vi "Add Sub Address.vi"(0 "Remote Terminal in":refnum<k24>, 1 "SubAddress Config":T1 {"elapseMinOrMax" items=["A", "B", "AB", "None"]; "timeOrHitCount" items=["Time", "HitCount"]; "dataWipe" items=["Simulate", "Monitor", "Disable"]}, 5 "name":string, 7 "subAddress":i8, 9 "messageBufferIDRef (-1)":i32=-1, 11 "error in":errorcluster, 12 "direction (Tx)":i32(ring) items=["Tx", "Rx"]) -> (4 "Remote Terminal out":refnum<k24>, 6 "new Sub Address":refnum<k24>, 8 "ID out":i32, 15 "error out":errorcluster)   [LabVIEW 2020, in "Ballard_1553_Hardware_ni.lvlib"]
uses:
  Ballard_1553_Hardware_ni.lvlib
  C:/Users/Administrator/Desktop/GIT/Ballard-MIL-STD-1553-Custom-Device/Source/System Explorer/SubVIs/Parse XML Ballard/1.2/BTIXML_SerDes.dll
  Ballard-MIL-STD-1553-Custom-Device/Source/System Explorer/SubVIs/Parse XML Ballard/1.2/BTIXML_SerDes.dll
  _typedefs/subAddress_type.ctl
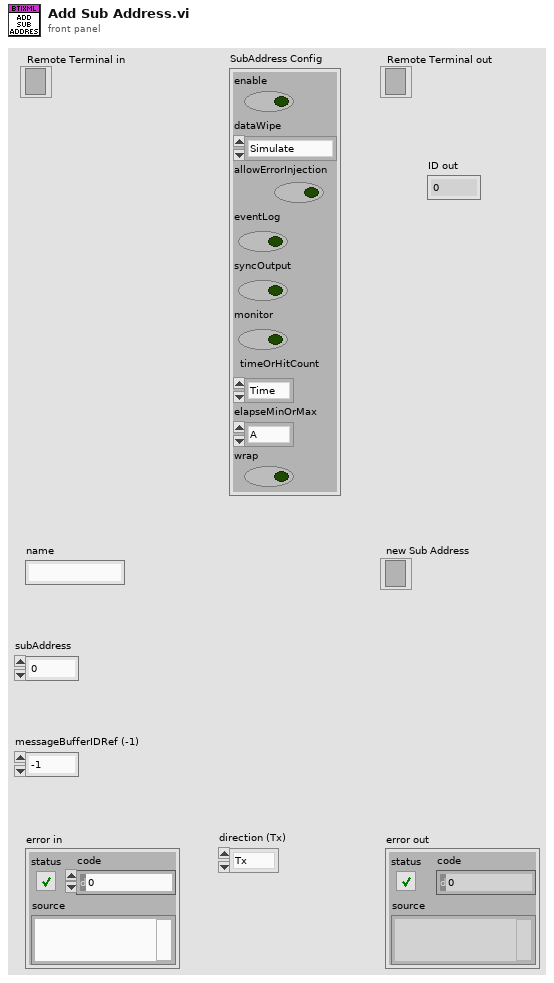
[diagram p1: front panel]
types:
  T1 = typedef "Ballard_1553_Hardware_ni.lvlib/subAddress_type.ctl" = cluster{"enable":bool, "dataWipe":i32, "allowErrorInjection":bool, "eventLog":bool, "syncOutput":bool, "monitor":bool, "timeOrHitCount":i32, "elapseMinOrMax":i32, "wrap":bool}
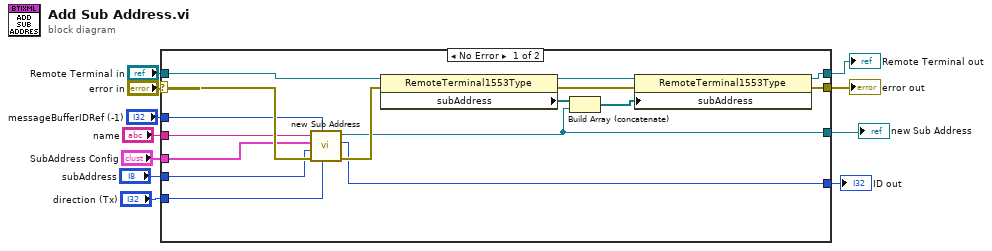
[diagram p0: block diagram]
diagram:
  n1 = case shown="No Error" "error in" {
    selector: "error in" -> [w20 w28]
    tunnel: [w25 w28] -> w11
    tunnel: [w26 w29] -> w8
    tunnel: "Remote Terminal in" -> [w27 w29]
    tunnel: [w18 _] -> w7
    tunnel: "messageBufferIDRef (-1)" -> [w17 _]
    tunnel: "name" -> [w16 _]
    tunnel: "SubAddress Config" -> [w15 _]
    tunnel: "direction (Tx)" -> [w14 _]
    tunnel: "subAddress" -> [w13 _]
    tunnel: [w12 _] -> w1
    frame No Error {
      n2 = call "new Sub Address.vi"("direction (Tx)"=w14, "messageBufferIDRef (-1)"=w17, "error in"=w20, "subAddress"=w13, "SubAddress Config"=w15, "name"=w16) -> ("error out"=w19:errorcluster, "ID out"=w12:i32, "subAddress out"=w18:refnum<k24>)  [unwired: 3 in]
      n3 = property class="RemoteTerminal1553Type"(reference=w27, error in=w19) -> (reference out=w21:refnum<k24>, error out=w22:errorcluster, "subAddress"=w24:refnum<k24>[])
      n4 = Build Array (concatenate)(w24, w18) -> (w23:refnum<k24>[])
      n5 = property class="RemoteTerminal1553Type"(reference=w21, error in=w22, "subAddress"=w23) -> (reference out=w26:refnum<k24>, error out=w25:errorcluster)
    }
    frame Error {
    }
  }
  "error out" <- w11
  "Remote Terminal out" <- w8
  "new Sub Address" <- w7
  "ID out" <- w1
